vi "Read Report Folder.vi"(8 "error in (no error)":errorcluster, 11 "Sequencer Module configuration in":refnum<class "Sequencer Module configuration.lvclass">) -> (0 "error out":errorcluster, 2 "Report Folder":string, 3 "Sequencer Module configuration out":refnum<class "Sequencer Module configuration.lvclass">)   [LabVIEW 2015, in "Sequencer Module configuration.lvclass"]
uses:
  Sequencer Module configuration.lvclass
  Sequencer Module configuration.lvclass/Sequencer Module configuration.ctl
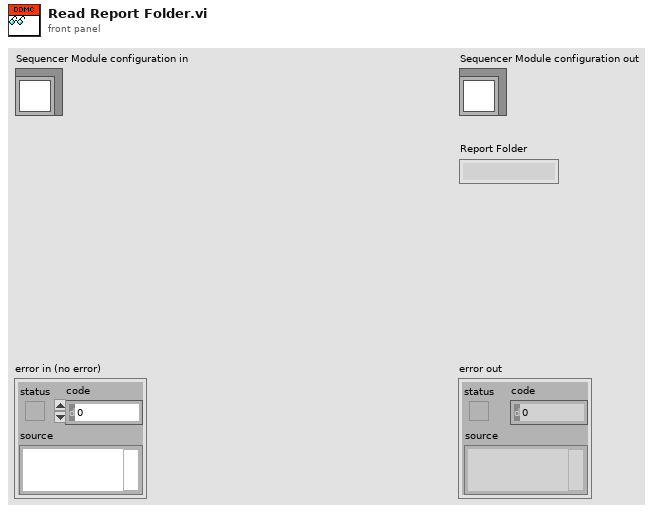
[diagram p1: front panel]
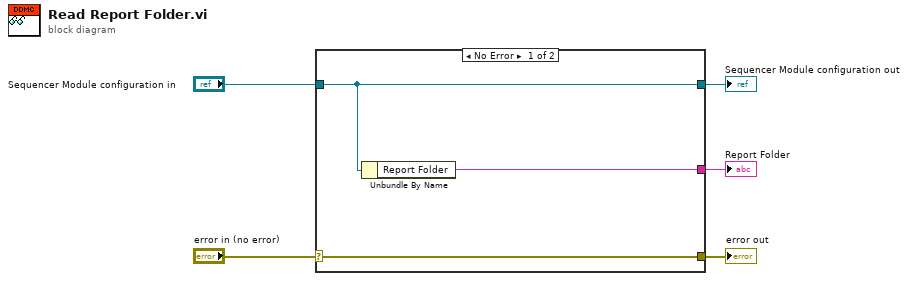
[diagram p0: block diagram]
diagram:
  n1 = case shown="No Error" "error in (no error)" {
    selector: "error in (no error)" -> [w8 w9]
    tunnel: [w8 w9] -> w4
    tunnel: [w7 w10] -> w2
    tunnel: "Sequencer Module configuration in" -> [w7 w10]
    tunnel: [w6 _] -> w1
    frame No Error {
      n2 = Unbundle By Name(w7) -> ("Report Folder"=w6:string)
    }
    frame Error {
    }
  }
  "error out" <- w4
  "Sequencer Module configuration out" <- w2
  "Report Folder" <- w1
